vi "Get Specified Objects.vi"(8 "error in":errorcluster, 9 "Secondary Data":string, 10 "Object Type":T1(ring)=enum."Generic", 11 "Diagram In":refnum<vi>) -> (0 "error out":errorcluster, 2 "All Objects":refnum<vi>[](array[refnum]), 3 "Diagram Out":refnum<vi>)   [LabVIEW 2018, in "Scripting Tools.lvlib"]
doc: "Returns all GObjects from the block diagram referenced by <B>Diagram In</B>, including all those in sub-diagrams (loops and sequence structures etc)."
uses:
  Scripting Tools.lvlib
  <vilib>/Utility/traverseref.llb/TRef TravTarget.ctl
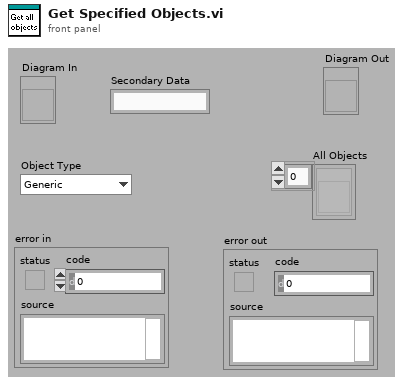
[diagram p1: front panel]
types:
  T1 = enum16{"Application", "VI", "PolymorphicVI", "MethodVI", "FacadeVI", "Generic", "FlatSequenceFrame", "TimeSequenceFrame", "SubWizard", "CodeWizard", "StateDiagramWizard", "MasterWizard", "Probe", "ConnectorPane", "Page", "Cursor", "Plot", "GObject", "TimedStructDCO", "SynchronousDataFlowDCO", "PolymorphicVISelector", "FlatSequenceOuterTunnel", "FlatSequenceInnerTunnel", "SimulationDCO", "FlatSequence", "TimeFlatSequence", "PropertyItem", "Wire", "SequenceLocal", "Tunnel", "SelectorTunnel", "LeftShiftRegister", "LoopTunnel", "RightShiftRegister", "Node", "TimedSequence", "XNode", "XDataNode", "StaticVIReference", "ControlReferenceConstant", "GrowableFunction", "Unbundler", "NamedUnbundler", "FormatScanString", "ObjectFunction", "Constructor", "Invoke", "Property", "CallLibrary", "CIN", "Bundler", "NamedBundler", "BuildArray", "IndexArray", "CompoundArithmetic", "BuildClusterArray", "Formula", "MathScriptNode", "ScriptNode", "Structure", "SynchronousDataFlowNode", "SimulationNode", "MultiFrameStructure", "DisableStructure", "EventStructure", "CaseStructure", "Sequence", "ExternalNode", "Loop", "WhileLoop", "TimedLoop", "ForLoop", "UnitCast", "CallByRef", "SubVI", "ConfNode", "PolymorphicSubVI", "Function", "FileDialog", "ArrayToCluster", "GPIBReadWrite", "FlattenUnflattenString", "FlattenString", "TypeCast", "ReadWriteFile", "Comparison", "Local", "Global", "FormulaParameter", "MathScriptNodeParameter", "ScriptNodeParameter", "Constant", "LabVIEWClassConstant", "AbsTimeConstant", "RefNumConstant", "ClassSpecifierConstant", "ColorBoxConstant", "IONameConstant", "GenClassTagFlatRefConstant", "GenClassTagRefConstant", "DAQmxNameConstant", "IVILogicalNameConstant", "VISAResourceNameConstant", "DAQChannelNameConstant", "DSCTagConstant", "BooleanConstant", "FixedConstant", "ClusterConstant", "StringConstant", "ComboBoxConstant", "NumericConstant", "NamedNumericConstant", "EnumConstant", "RingConstant", "DigitalNumericConstant", "ArrayConstant", "PathConstant", "Terminal", "OuterTerminal", "InnerTerminal", "ControlTerminal", "AbstractDiagram", "MathDiagram", "Diagram", "SDFCompanionDiagram", "SdfDiagram", "CompanionDiagram", "SimDiagram", "TopLevelDiagram", "Splitter", "Pane", "Scale", "SlideScale", "ColorGraphScale", "GraphScale", "ColorScale", "RotaryColorScale", "Panel", "Control", "LabVIEWClassControl", "SceneGraphDisplay", "Scrollbar", "Pixmap", "PlugInDDODummyContainer", "PlugInControl", "TreeControl", "SubPanel", "DigitalTable", "AbsTime", "PageSelector", "TabControl", "WaveformData", "MulticolumnListbox", "Cluster", "RadioButtonsControl", "IOName", "GenClassTagFlatRef", "GenClassTagRef", "DAQmxName", "IVILogicalName", "VISAResourceName", "DAQChannelName", "DSCTag", "String", "ComboBox", "GraphChart", "MixedSignalGraph", "IntensityGraph", "IntensityChart", "WaveformGraph", "DigitalGraph", "XYGraph", "WaveformChart", "Numeric", "NumericWithScale", "Knob", "Slide", "ColorRamp", "NamedNumeric", "Enum", "Ring", "Digital", "ActiveXContainer", "Picture", "Array", "Table", "ListBox", "Path", "LVVariant", "RefNum", "GenClassRef", "LVObjectRefNum", "VIRefNum", "TypedRefNum", "Boolean", "ColorBox", "Decoration", "Text", "NumericText", "Project", "ProjectItem", "PropertyFolder", "XPropertyFolder", "TargetItem", "Library", "XInterfaceLibrary", "XNodeLibrary", "XControlLibrary", "LVClassLibrary", "BuildSpecification", "Variable", "TagSet", "SceneWindow", "LVTarget", "Provider", "CopyOperation", "ProjectItemType", "CopyItem", "CopyConflict", "CopyExpert", "SceneNode", "SceneClipPlane", "SceneLight", "SceneObject", "SceneTexture", "SceneGeometry", "SceneMesh", "SceneSphere", "SceneHeightField", "SceneCylinder", "SceneCone", "SceneBox"}
  T2 = typedef "TRef TravTarget.ctl" = enum16{"FP", "BD", "Other"}
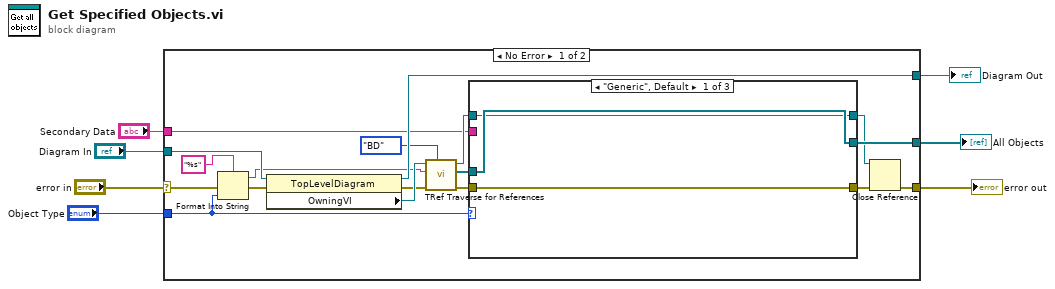
[diagram p0: block diagram]
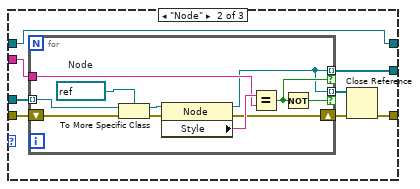
[diagram p2: hidden frame]
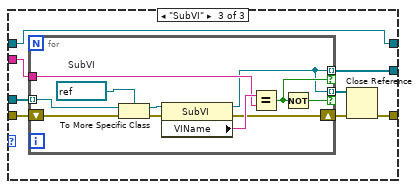
[diagram p3: hidden frame]
diagram:
  n1 = case shown="No Error" "error in" {
    selector: "error in" -> [w9 w68]
    tunnel: [w22 w68] -> w7
    tunnel: "Diagram In" -> [w25 w67]
    tunnel: [w21 w67] -> w5
    tunnel: [w18 _] -> w3
    tunnel: "Secondary Data" -> [w13 _]
    tunnel: "Object Type" -> [w12 _]
    frame No Error {
      n2 = Format Into String(format string="%s", error in=w9, w12) -> (resulting string=w10:string, error out=w8:errorcluster)  [unwired: 1 in]
      n3 = property on="Property Node" class="TopLevelDiagram"(reference=w25, error in=w8) -> (reference out=w21:refnum<vi>, error out=w23:errorcluster, "OwningVI"=w24:refnum<vi>)
      n4 = call <vilib>:"TRef Traverse for References.vi"("Traverse Target"=TRef_TravTarget."BD", "error in (no error)"=w23, "Class Name"=w10, "VI Refnum"=w24) -> ("error out"=w14:errorcluster, "References"=w19:refnum<vi>[], "dup VI Refnum"=w16:refnum<vi>)  [unwired: 1 in, 4 out]
      n5 = case shown="\"Generic\", Default" w12 {
        tunnel: w19 -> [w28 w36 w55]
        tunnel: [w28 w33 w52] -> w18
        tunnel: [w27 w32 w51] -> w17
        tunnel: w16 -> [w27 w32 w51]
        tunnel: [w26 w31 w50] -> w15
        tunnel: w14 -> [w26 w35 w54]
        tunnel: w13 -> [_ w34 w53]
        frame "Generic", Default {
        }
        frame "Node" {
          n6 = for {
            tunnel: w36 -> [w47] mode=indexing
            shift-right: [w37] -> w29
            shift-left: w35 -> [w43]
            tunnel: w34 -> [w41]
            tunnel: [w39] -> w33 mode=indexing if=w40
            tunnel: [w39] -> w30 mode=indexing if=w38
            w46 = refnum<vi> refnum  # Node
            n7 = To More Specific Class(target class=w46, reference=w47, error in=w43) -> (specific class reference=w45:refnum<vi>, error out=w44:errorcluster)
            n8 = property class="Node"(reference=w45, error in=w44) -> (reference out=w39:refnum<vi>, error out=w37:errorcluster, "Style"=w42:string)
            n9 = Equal?(x=w42, y=w41) -> (x = y?=w40:bool)
            n10 = Not(x=w40) -> (.not. x?=w38:bool)
          }
          n11 = Close Reference(reference=w30, error in (no error)=w29) -> (error out=w31:errorcluster)
        }
        frame "SubVI" {
          n12 = for {
            tunnel: w55 -> [w66] mode=indexing
            shift-right: [w56] -> w48
            shift-left: w54 -> [w62]
            tunnel: w53 -> [w60]
            tunnel: [w58] -> w52 mode=indexing if=w59
            tunnel: [w58] -> w49 mode=indexing if=w57
            w65 = refnum<vi> refnum  # SubVI
            n13 = To More Specific Class(target class=w65, reference=w66, error in=w62) -> (specific class reference=w64:refnum<vi>, error out=w63:errorcluster)
            n14 = property class="SubVI"(reference=w64, error in=w63) -> (reference out=w58:refnum<vi>, error out=w56:errorcluster, "VIName"=w61:string)
            n15 = Equal?(x=w61, y=w60) -> (x = y?=w59:bool)
            n16 = Not(x=w59) -> (.not. x?=w57:bool)
          }
          n17 = Close Reference(reference=w49, error in (no error)=w48) -> (error out=w50:errorcluster)
        }
      }
      n18 = Close Reference(reference=w17, error in (no error)=w15) -> (error out=w22:errorcluster)
    }
    frame Error {
    }
  }
  "error out" <- w7
  "All Objects" <- w3
  "Diagram Out" <- w5
